vi "GetID.vi"(8 "error in (no error)":errorcluster, 11 "reference in":refnum<class "Laser.lvclass">) -> (0 "error out":errorcluster, 2 "Id String":string, 3 "reference in":refnum<class "Laser.lvclass">)   [LabVIEW 2012]
uses:
  Laser.lvclass
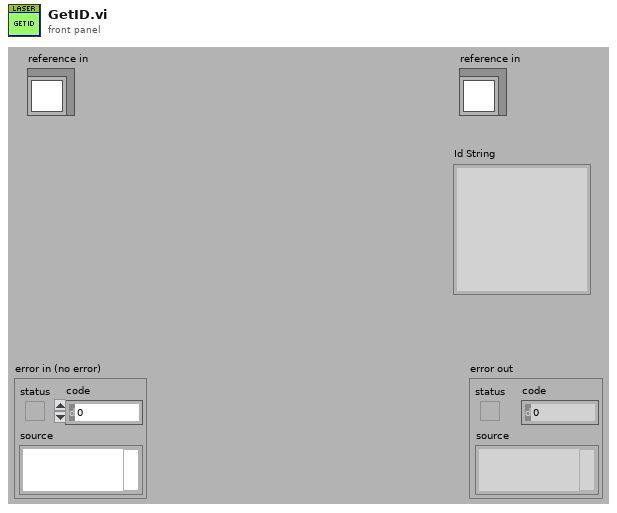
[diagram p1: front panel]
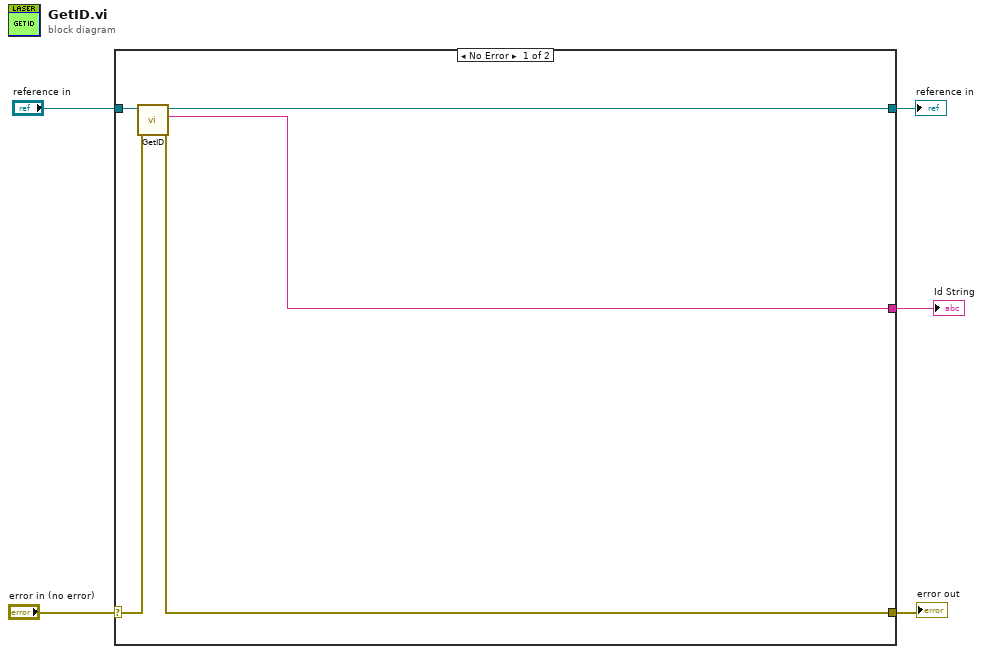
[diagram p0: block diagram]
diagram:
  n1 = case shown="No Error" "error in (no error)" {
    selector: "error in (no error)" -> [w10 w12]
    tunnel: [w7 w12] -> w4
    tunnel: [w8 w11] -> w2
    tunnel: "reference in" -> [w9 w11]
    tunnel: [w6 _] -> w1
    frame No Error {
      n2 = call-dynamic "GetID.vi"("error in (no error)"=w10, "reference in"=w9) -> ("error out"=w7:errorcluster, "Id String"=w6:string, "reference out"=w8:refnum<class "Laser.lvclass">)  [unwired: 7 in]
    }
    frame Error {
    }
  }
  "error out" <- w4
  "reference in" <- w2
  "Id String" <- w1
